vi "Source Status query.vi"(8 "error in (no error)":errorcluster, 11 "VISA resource name":refnum<visa-resource-name>) -> (0 "error out":errorcluster, 2 "Status":string, 3 "VISA resource name out":refnum<visa-resource-name>)   [LabVIEW 2025, in "Chroma 19052.lvlib"]
doc: "Chroma\n5 Clock Tower Place Suite 210\nMaynard, MA 01754\nTel: 1 800 253-1230\nTel: 1 877 4 A HIPOT\nFax: 1 978-461-4295\nWebsite: www.chroma.com"
uses:
  <instrlib>/Chroma 19052/Chroma 19052.lvlib
  <vilib>/Utility/error.llb/Trim Whitespace One-Sided.vi
panel:
  # "Execution Status query"
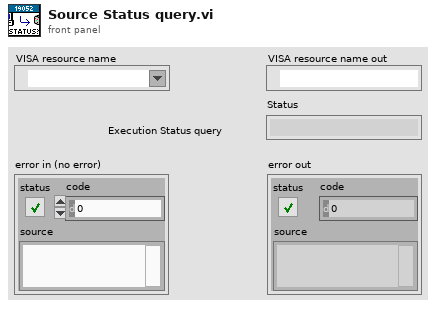
[diagram p1: front panel]
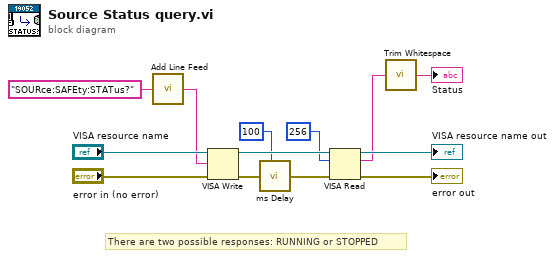
[diagram p0: block diagram]
diagram:
  # "There are two possible responses: RUNNING or STOPPED"
  n1 = call <instrlib>:"Add Line Feed.vi"("Command string"="SOURce:SAFEty:STATus?") -> ("Concatenated string"=w8:string)  [unwired: 4 in]
  n2 = VISA Write(VISA resource name="VISA resource name", write buffer=w8, error in (no error)="error in (no error)") -> (VISA resource name out=w13:refnum<visa-resource-name>, error out=w5:errorcluster)  [unwired: 1 out]
  n3 = call <instrlib>:"ms Delay.vi"("miliseconds to wait"=u32 100 ("Time Delay ms"), "error in (no error)"=w5) -> ("error out"=w4:errorcluster)  [unwired: 6 in, 1 out]
  n4 = VISA Read(VISA resource name=w13, byte count=u32 256, error in (no error)=w4) -> (VISA resource name out=→"VISA resource name out":refnum<visa-resource-name>, read buffer=w2:string, error out=→"error out":errorcluster)  [unwired: 1 out]
  n5 = call <vilib>:"Trim Whitespace.vi"("string"=w2) -> ("trimmed string"=→"Status":string)  [unwired: 1 in]
